vi "Receive Message.vi"(8 "error in (no error)":errorcluster, 9 "Mail Strategy In":refnum<class "Mail Strategy.lvclass">, 10 "Wait(ms)":i32=-1, 11 "Map Tree Queue Messenger Component in":refnum<class "Map Tree Queue Messenger.lvclass">) -> (0 "error out":errorcluster, 1 "Valid":bool, 2 "Message Out":refnum<class "Message.lvclass">, 3 "Map Tree Queue Messenger Component out":refnum<class "Map Tree Queue Messenger.lvclass">)   [LabVIEW 2019, in "Map Tree Queue Messenger.lvclass"]
uses:
  Map Tree Queue Messenger.lvclass
  C:/Users/iio/Desktop/Bussiness/MultiSPIM/General Library/Ancestor Class/Messenger/Messenger Map Composite/Messenger Map Composite.lvclass
  Ancestor Class/Message/Message.lvclass
  Ancestor Class/Messenger/Mail Strategy/Mail Strategy.lvclass
  Simple Tree Queue Mailman/Simple Tree Queue Mailman.lvclass
  C:/Users/iio/Desktop/Bussiness/MultiSPIM/General Library/Ancestor Class/Messenger/Mail Strategy/Mail Strategy.lvclass
  Ancestor Class/Messenger/Messenger Map Composite/Messenger Map Composite.lvclass/Messenger Map Composite.ctl
  Simple Tree Queue Mailman/Simple Tree Queue Mailman.lvclass/Simple Tree Queue Mailman.ctl
  Map Tree Queue Messenger.lvclass/Map Tree Queue Messenger.ctl
  Simple Tree Queue Mailman/Public Data/Write Address Recursive Access.vi
  Ancestor Class/Messenger/Messenger Map Composite/Public Data/Read Child Nodes.vi
  Ancestor Class/Messenger/Messenger/Messenger.lvclass
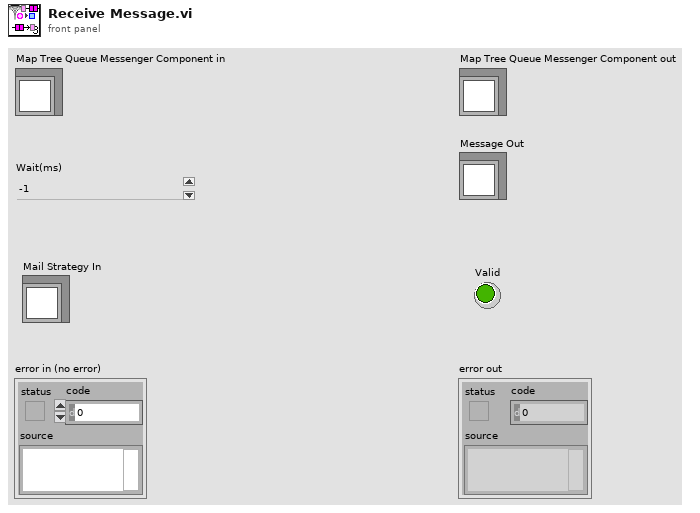
[diagram p1: front panel]
types:
  T1 = typedef "Message Queue.ctl" = refnum<queue>
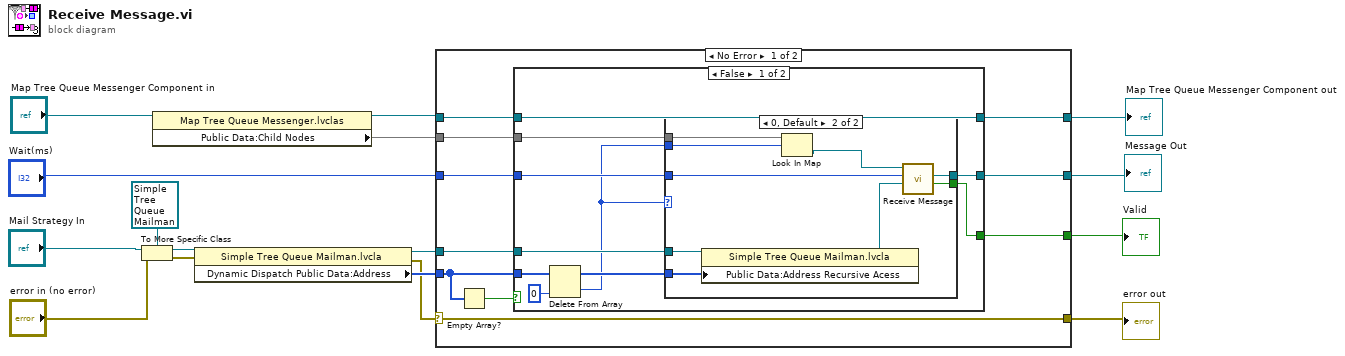
[diagram p0: block diagram]
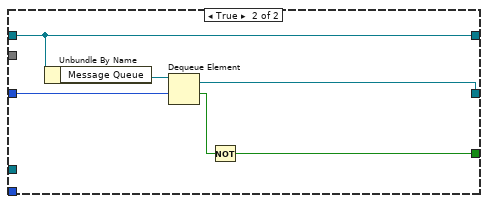
[diagram p3: hidden frame]
diagram:
  n1 = To More Specific Class(target class=refnum<class "Simple Tree Queue Mailman.lvclass"> refnum ("Array Location Mailman.lvclass"), reference="Mail Strategy In", error in="error in (no error)") -> (specific class reference=w15:refnum<class "Simple Tree Queue Mailman.lvclass">, error out=w16:errorcluster)
  n2 = property class="Map Tree Queue Messenger.lvclas"(reference="Map Tree Queue Messenger Component in") -> (reference out=w11:refnum<class "Map Tree Queue Messenger.lvclass">, "Public Data:Child Nodes"=w10:map{i64, refnum<class "Messenger.lvclass">})  [unwired: 1 in, 1 out]
  n3 = property class="Simple Tree Queue Mailman.lvcla"(reference=w15, error in=w16) -> (reference out=w12:refnum<class "Simple Tree Queue Mailman.lvclass">, error out=w13:errorcluster, "Dynamic Dispatch Public Data:Address"=w14:i32[])
  n4 = case shown="No Error" w13 {
    selector: w13 -> [w24 w53]
    tunnel: w11 -> [w23 w52]
    tunnel: "Wait(ms)" -> [w26 _]
    tunnel: [w25 _] -> w3
    tunnel: [w24 w53] -> w5
    tunnel: [w20 w52] -> w1
    tunnel: [w22 _] -> w4
    tunnel: w14 -> [w19 _]
    tunnel: w12 -> [w18 _]
    tunnel: w10 -> [w17 _]
    frame No Error {
      n5 = Empty Array?(array=w19) -> (empty?=w21:bool)
      n6 = case shown="False" w21 {
        tunnel: w26 -> [w33 w50]
        tunnel: [w32 w49] -> w25
        tunnel: w23 -> [w34 w46]
        tunnel: [w31 w47] -> w22
        tunnel: [w34 w46] -> w20
        tunnel: w19 -> [w36 _]
        tunnel: w18 -> [w30 _]
        tunnel: w17 -> [w28 _]
        frame False {
          n7 = Delete From Array(array=w36, index=0) -> (deleted portion=w27:i32, array with subset deleted=w29:i32[])  [unwired: 1 in]
          n8 = case shown="0, Default" w27 {
            tunnel: w33 -> [_ w45]
            tunnel: [_ w44] -> w32
            tunnel: [_ w43] -> w31
            tunnel: w27 -> [_ w38]
            tunnel: w30 -> [_ w42]
            tunnel: w29 -> [_ w41]
            tunnel: w28 -> [_ w39]
            frame -2147483648..-1 {
            }
            frame 0, Default {
              n9 = property class="Simple Tree Queue Mailman.lvcla"(reference=w42, "Public Data:Address Recursive Acess"=w41) -> (reference out=w40:refnum<class "Simple Tree Queue Mailman.lvclass">)  [unwired: 1 in, 1 out]
              n10 = Look In Map(map=w39, key=w38) -> (value=w37:refnum<class "Messenger.lvclass">)  [unwired: 1 in, 1 out]
              n11 = call-dynamic "Receive Message.vi"("Mail Strategy In"=w40, "Wait(ms)"=w45, "Messenger Component in"=w37) -> ("Valid"=w43:bool, "Message Out"=w44:refnum<class "Message.lvclass">)  [unwired: 5 in, 2 out]
            }
          }
        }
        frame True {
          n12 = Unbundle By Name(w46) -> ("Message Queue"=w51:T1)
          n13 = Dequeue Element(queue=w51, timeout in ms (-1)=w50) -> (element=w49:refnum<class "Message.lvclass">, timed out?=w48:bool)  [unwired: 1 in, 2 out]
          n14 = Not(x=w48) -> (.not. x?=w47:bool)
        }
      }
    }
    frame Error {
    }
  }
  "error out" <- w5
  "Map Tree Queue Messenger Component out" <- w1
  "Message Out" <- w3
  "Valid" <- w4
